vi "Auto Intake Mode.vi"(7 "Intake Angle":dbl, 11 "Intake Commands Cluster":T2={"Intake Commands"=enum."Load", "Intake Mode"=enum."Auto", "Override IR"=FALSE}) -> (0 "Intake States":T1, 2 "Roller Power":dbl, 3 "Angle Power":dbl, 4 "Target Height":dbl, 5 "Encoder Position":dbl, 6 "Rollers Active?":bool)   [LabVIEW 2015]
uses:
  Common Code/Intake Commands Cluster.ctl
  Common Code/Intake Commands.ctl
  Common Code/Intake Mode.ctl
  Common Code/Intake States.ctl
  Common Code/Change Detect Int.vi
  Common Code/Change Detect Double.vi
  Robot Global Data.vi
  <vilib>/addons/control/pid/pid.llb/PID (DBL).vi
  <vilib>/addons/control/pid/NI_PID_pid.lvlib
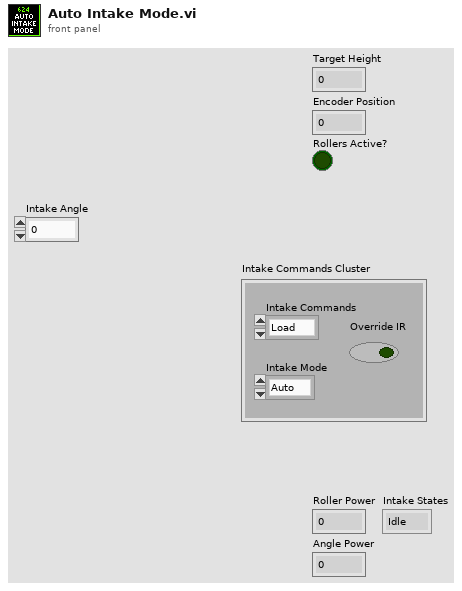
[diagram p1: front panel]
types:
  T1 = typedef "Intake States.ctl" = enum16{"Idle", "Set roller speed", "Move to angle"}
  T2 = typedef "Intake Commands Cluster.ctl" = cluster{"Intake Commands":T3, "Intake Mode":T4, "Override IR":bool}
  T3 = typedef "Intake Commands.ctl" = enum16{"Unload", "Load", "Pull up", "Drop low", "Idle", "Lift Half"}
  T4 = typedef "Intake Mode.ctl" = enum16{"Safe", "Auto", "Manual"}
  T5 = typedef "Dashboard Control Data.ctl" = cluster{"Shooter Presets":T6, "Encoder Control":T8, "Steer PID output":cluster{"output high":dbl, "output low":dbl}, " Steer PID gains":cluster{"proportional gain (Kc)":dbl, "integral time (Ti, min)":dbl, "derivative time (Td, min)":dbl}, "Drivetrain Settings":T9, "Vision Packet":T10, "Dashboard Drivetrain Command":T11, "Info/Command Cluster":T13, "Ball Vision Packet":T14, "Intake Presets":T16, "Intake Encoder Control":T18, "Climb Presets":T19, "Goal Output Range":cluster{"output high":dbl, "output low":dbl}, "Enabled Systems":T20, "Auton Presets":T21, "Pressure M":dbl, "Pressure B":dbl}
  T6 = typedef "Shooter Presets.ctl" = cluster{"Batter Shot":T7, "Deep Middle Shot":T7, "Manual Shot":T7, "Left Ticks Per Rotation":dbl, "Right Ticks Per Rotation":dbl, "Low Bar Shot":T7, "Shooter RPM Tolerance":dbl, "IIR Filter Power":dbl, "Trigger Power":dbl, "Fire from Load Delay":i32, "Max Angle":dbl, "Min Angle":dbl, "Angle PID gains":cluster{"P":dbl, "I":dbl, "D":dbl}, "Angle Output":cluster{"output high":dbl, "output low":dbl}, "Shooter Angle Tolerance":dbl, "Vision Shoot x^2":dbl, "Vision Shoot x":dbl, "Axis Camera Offset":dbl, "High Goal Center Height":dbl, "Feed Forward Max Accel":dbl, "Feed Forward Kv":dbl, "Backwards Trigger":dbl, "Shot Finish Delay (ms)":dbl, "Angle Max Current":dbl, "Angle Current Trip Time":dbl, "Intake Angle":dbl, "Vision Shoot c":dbl, "Reset?":bool, "Servo Release Delay":dbl, "Servo Idle Angle":i32, "Servo Hold Angle":i32, "Angle Pot x":dbl, "Angle Pot c":dbl, "Ignore Angle?":bool, "Manual Output?":bool, "Manual Out":dbl, "Max RPM":dbl, "Safty Frist Angle":dbl, "Intake Danger Height":dbl, "Angle Pot B":i32, "Angle Pot M":dbl, "FF Finish RPM":dbl, "RPM PID Right":cluster{"P":dbl, "I":dbl, "D":dbl, "FF":dbl}, "RPM PID Left":cluster{"P":dbl, "I":dbl, "D":dbl, "FF":dbl}, "Backwards RPM":dbl, "Vision RPM":dbl}
  T7 = typedef "Shot Presets.ctl" = cluster{"Left":dbl, "Right":dbl, "Angle":dbl}
  T8 = typedef "Encoder Control.ctl" = cluster{"Right Tick Constant":dbl, "Left Tick Constant":dbl, "Reset?":bool, "Y Dist":cluster{"PID gains":cluster{"proportional gain (Kc)":dbl, "integral time (Ti, min)":dbl, "derivative time (Td, min)":dbl}}, "Y Stop Thresh":dbl, "Y Stop Speed":dbl}
  T9 = typedef "Drivetrain Settings.ctl" = cluster{"Gyro Tolerance":dbl, "Throttle Ramp (ms)":dbl, "Angular rate compensation":bool, "Throttle to Rate Scale":dbl, "Rate compensation gain":dbl, "Kv":dbl, "Ka":dbl, "Feed Forward P":dbl, "Feed Forward D":dbl, "Goal Vision PID gains":cluster{"proportional gain (Kc)":dbl, "integral time (Ti, min)":dbl, "derivative time (Td, min)":dbl}, "Goal Detection Window":dbl, "Creep Rate":dbl}
  T10 = typedef "Goal Vision Packet.ctl" = cluster{"Distance":dbl, "Center X":dbl, "Center Y":dbl, "Found Target?":bool, "Robot Center":dbl, "Angle":dbl}
  T11 = typedef "Dashboard Drivetrain Command.ctl" = cluster{"Drivetrain Vision":T12}
  T12 = typedef "Drivetrain Vision.ctl" = cluster{"Goal Window":dbl, "Ball Window":dbl}
  T13 = typedef "Ball Tracking Command Cluster.ctl" = cluster{"Distance to Ball":dbl, "Desired Angle":dbl, "Command":enum16{"Turn to Ball", "Turn to Angle", "Get Distance"}, "Pixels from Center":dbl}
  T14 = typedef "Ball Vision Packet.ctl" = cluster{"Ball Detected?":bool, "Distance to Ball":dbl, "Desired Angle":dbl, "Pixels from Center":dbl, "Tracking mode":T15}
  T15 = typedef "Tracking Mode.ctl" = enum16{"Turn to Ball", "Turn to Angle"}
  T16 = typedef "Intake Presets.ctl" = cluster{"Intake Speed":dbl, "Outake Speed":dbl, "Low Height":dbl, "Half Height":dbl, "Full Height":dbl, "Angle Speed":dbl, "Angle Tolerance":dbl, "Encoder Scale":dbl, "Load Height":dbl, "Output Range":T17, "Rotation Power Max/Min":dbl, "MaxCurrent":dbl, "Intake Trip Time":dbl, "Idle Height":dbl, "Max Height":dbl, "Reset Encoders?":bool, "PID gains":cluster{"proportional gain (Kc)":dbl, "integral time (Ti, min)":dbl, "derivative time (Td, min)":dbl}}
  T17 = typedef "Drivetrain Output Range.ctl" = cluster{"output high":dbl, "output low":dbl}
  T18 = typedef "IntakeEcoderControl.ctl" = cluster{"Arm Tick Constant":dbl, "Reset?":bool, "Y Dist":cluster{"PID gains":cluster{"proportional gain (Kc)":dbl, "integral time (Ti, min)":dbl, "derivative time (Td, min)":dbl}}, "Y Stop Thresh":dbl, "Y Stop Speed":dbl}
  T19 = typedef "Climb Presets.ctl" = cluster{"Pull Power":dbl, "Time to Hold":dbl, "Extend Power":dbl}
  T20 = typedef "Enabled Systems.ctl" = cluster{"Shoot":bool, "Intake":bool, "DT":bool, "Gyro":bool, "100ms":bool, "US":bool}
  T21 = typedef "Autonomous Presets.ctl" = cluster{"Pitch Limit":dbl, "Roll Limit":dbl, "Ultrasonic Limit":dbl, "Start Position":dbl, "Cross Position":dbl}
  T22 = cluster{"proportional gain (Kc)":dbl, "integral time (Ti, min)":dbl, "derivative time (Td, min)":dbl}
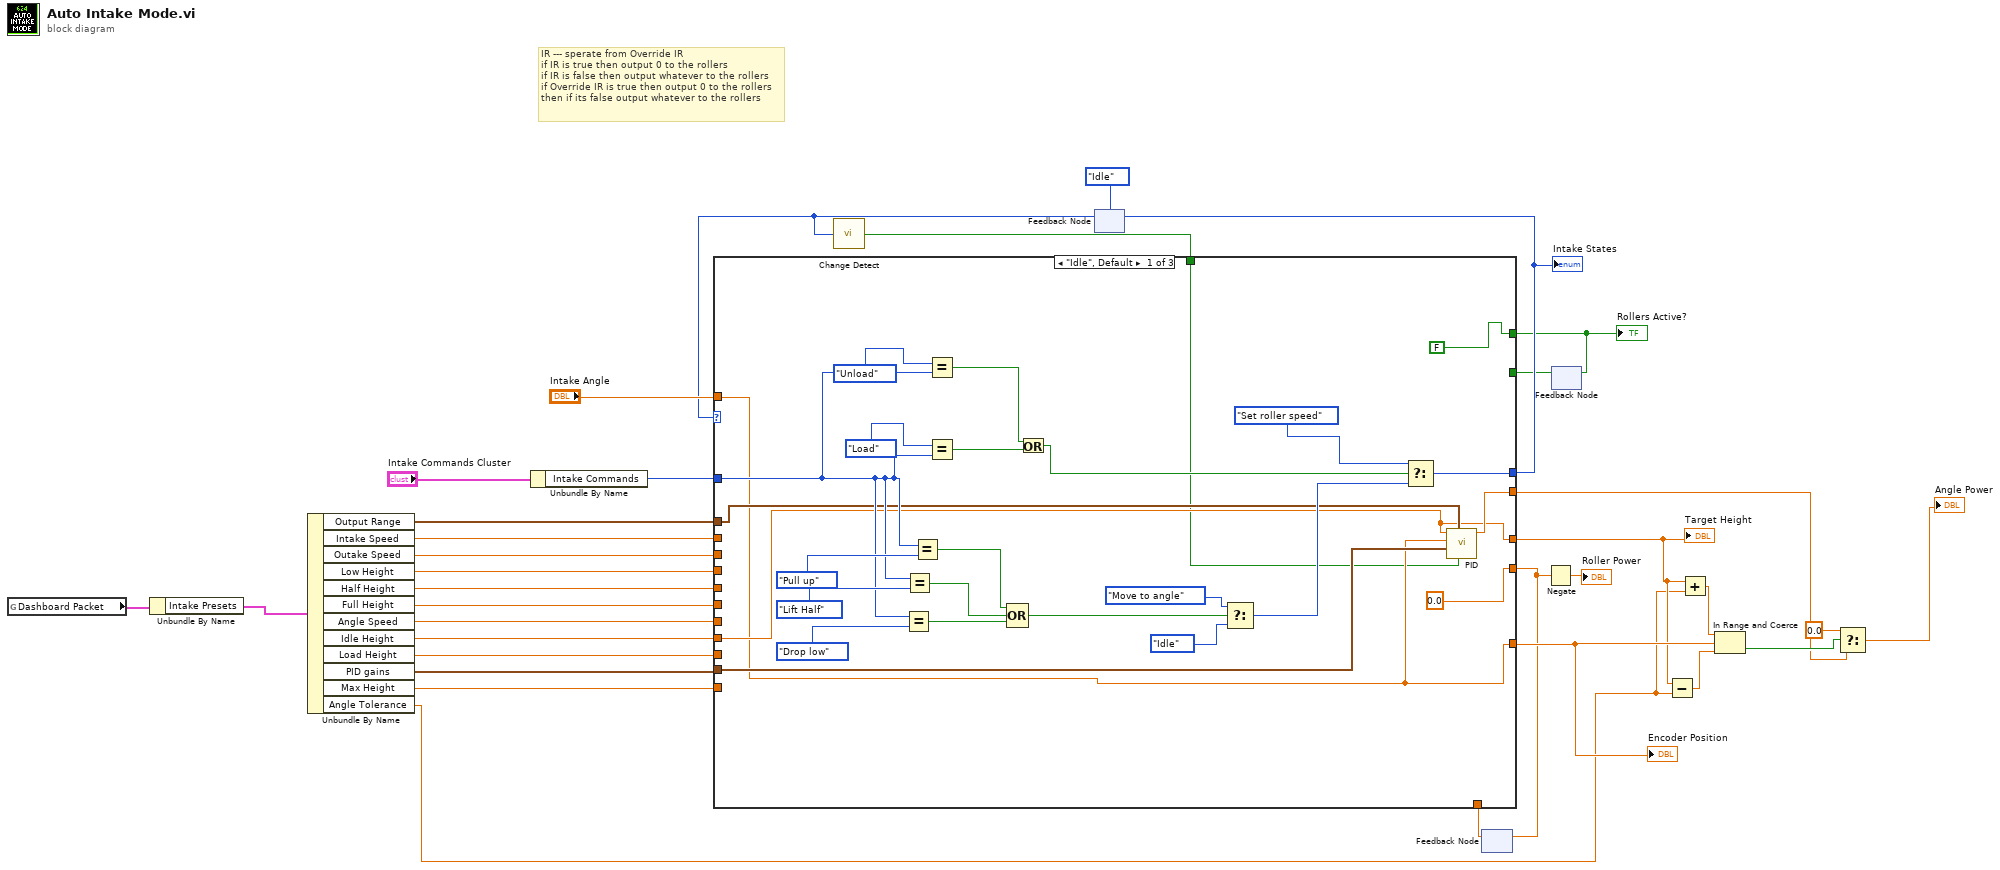
[diagram p0: block diagram]
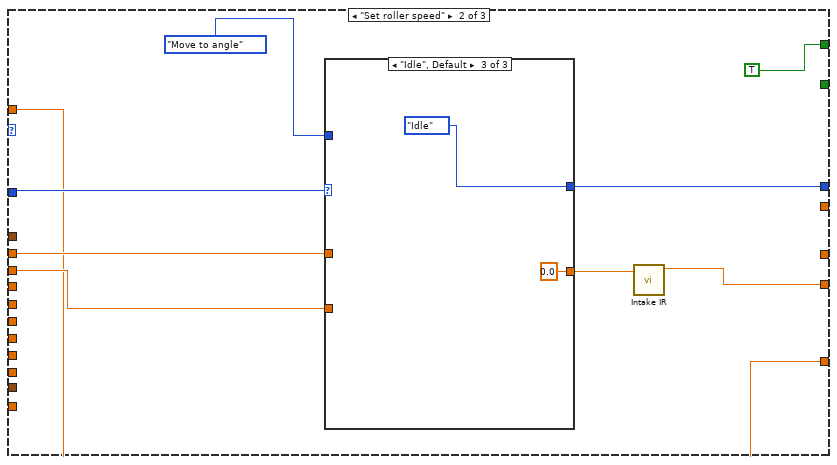
[diagram p2: hidden frame]
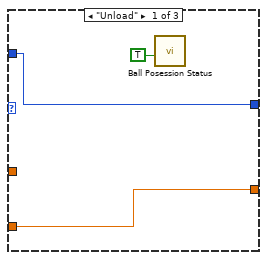
[diagram p3: hidden frame]
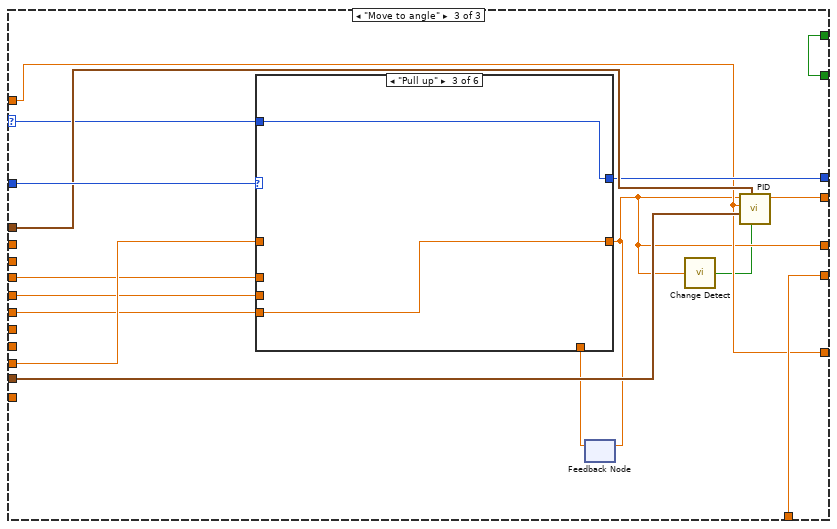
[diagram p5: hidden frame]
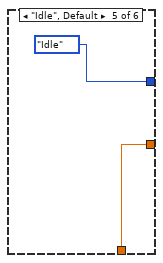
[diagram p9: hidden frame]
diagram:
  # "IR --- sperate from Override IR \nif IR is true then output 0 to the rollers\nif IR is false then output whatever to the rollers\nif Override IR is true then output 0 to the rollers\nthen if its false output whatever to the rollers"
  n1 = global read "Robot Global Data.vi" "Dashboard Packet"() -> (w16:T5)
  n2 = Unbundle By Name(w16) -> ("Intake Presets"=w17:T16)
  n3 = Unbundle By Name(w17) -> ("Output Range"=w27:T17, "Intake Speed"=w26:dbl, "Outake Speed"=w25:dbl, "Low Height"=w24:dbl, "Half Height"=w23:dbl, "Full Height"=w22:dbl, "Angle Speed"=w21:dbl, "Idle Height"=w20:dbl, "Load Height"=w19:dbl, "PID gains"=w18:T22, "Max Height"=w15:dbl, "Angle Tolerance"=w12:dbl)
  n4 = Unbundle By Name("Intake Commands Cluster") -> ("Intake Commands"=w32:T3)
  n5 = feedback #1(Intake_States."Idle") -> (w5:T1)
  n6 = call-poly "Change Detect.vi"("In"=w5) -> ("Changed?"=w4:bool)
  n7 = feedback #2() -> (w30:dbl)  [unwired: 1 in]
  n8 = feedback #3() -> (w28:bool)  [unwired: 1 in]
  n9 = case shown="\"Idle\", Default" w5 {
    selector: w5 -> [_ _ w80]
    tunnel: w32 -> [w46 w69 w92]
    tunnel: [w50 w67 w81] -> w31
    tunnel: w27 -> [w40 _ w84]
    tunnel: w25 -> [_ w65 _]
    tunnel: w22 -> [_ _ w87]
    tunnel: w26 -> [_ w66 _]
    tunnel: w23 -> [_ _ w89]
    tunnel: w21 -> [_ _ _]
    tunnel: w24 -> [_ _ w88]
    tunnel: [0.0 ("Intake Speed") w63 w91] -> w3
    tunnel: w30 -> [_ _ w91]
    tunnel: w19 -> [_ _ w90]
    tunnel: [w39 _ w86] -> w1
    tunnel: "Intake Angle" -> [w36 w61 w79]
    tunnel: w18 -> [w41 _ w85]
    tunnel: w20 -> [w38 _ _]
    tunnel: [w38 _ w78] -> w13
    tunnel: [w36 w61 w79] -> w14
    tunnel: [FALSE TRUE w82] -> w29
    tunnel: w28 -> [_ _ w82]
    tunnel: w15 -> [_ _ _]
    tunnel: w4 -> [w35 _ _]
    frame "Idle", Default {
      n10 = Equal?(x=w46, y=Intake_Commands."Drop low" ("Intake Commands")) -> (x = y?=w52:bool)
      n11 = Equal?(x=w46, y=Intake_Commands."Lift Half" ("Intake Commands")) -> (x = y?=w53:bool)
      n12 = Equal?(x=w46, y=Intake_Commands."Pull up" ("Intake Commands")) -> (x = y?=w57:bool)
      n13 = Equal?(x=Intake_Commands."Unload" ("Intake Commands"), y=w46) -> (x = y?=w45:bool)
      n14 = Equal?(x=Intake_Commands."Load" ("Intake Commands"), y=w46) -> (x = y?=w44:bool)
      n15 = Compound Arithmetic op=OR(w57, w53, w52) -> (w56:bool)
      n16 = Or(x=w45, y=w44) -> (x .or. y?=w43:bool)
      n17 = Select(t=Intake_States."Move to angle", s=w56, f=Intake_States."Idle") -> (s? t:f=w51:T1)
      n18 = Select(t=Intake_States."Set roller speed", s=w43, f=w51) -> (s? t:f=w50:T1)
      n19 = call-poly <vilib>:"PID.vi"("reinitialize? (F)"=w35, "output range"=w40, "PID gains"=w41, "process variable"=w36, "setpoint"=w38) -> ("output"=w39:dbl)  [unwired: 5 in, 1 out]
    }
    frame "Set roller speed" {
      n20 = case shown="\"Idle\", Default" w69 {
        tunnel: Intake_States."Move to angle" -> [w72 w74 _]
        tunnel: [w72 w74 Intake_States."Idle"] -> w67
        tunnel: w66 -> [_ w73 _]
        tunnel: [w71 w73 0.0 ("Intake Speed")] -> w62
        tunnel: w65 -> [w71 _ _]
        frame "Unload" {
          n21 = call "Ball Posession Status.vi"("Logical Exit?"=TRUE) -> ()  [unwired: 10 in, 1 out]
        }
        frame "Load" {
        }
        frame "Idle", Default {
        }
      }
      n22 = call "Intake IR.vi"("Speed"=w62) -> ("Speeeeeeed"=w63:dbl)  [unwired: 10 in]
    }
    frame "Move to angle" {
      n23 = feedback #4() -> (w83:dbl)  [unwired: 1 in]
      n24 = case shown="\"Pull up\"" w92 {
        tunnel: w90 -> [w94 w96 _ _ _ _]
        tunnel: [w94 w96 w98 w100 w102 w104] -> w78
        tunnel: w89 -> [_ _ _ _ _ w104]
        tunnel: w88 -> [_ _ _ w100 _ _]
        tunnel: w87 -> [_ _ w98 _ _ _]
        tunnel: w83 -> [_ _ _ _ w102 _]
        tunnel: [w93 w95 w97 w99 Intake_States."Idle" w103] -> w81
        tunnel: w80 -> [w93 w95 w97 w99 _ w103]
        frame "Unload" {
        }
        frame "Load" {
        }
        frame "Pull up" {
        }
        frame "Drop low" {
        }
        frame "Idle", Default {
        }
        frame "Lift Half" {
        }
      }
      n25 = feedback-in #4(w78) -> ()
      n26 = call-poly "Change Detect.vi"("In"=w78) -> ("Changed?"=w77:bool)
      n27 = call-poly <vilib>:"PID.vi"("reinitialize? (F)"=w77, "output range"=w84, "PID gains"=w85, "process variable"=w79, "setpoint"=w78) -> ("output"=w86:dbl)  [unwired: 5 in, 1 out]
    }
  }
  "Intake States" <- w31
  "Target Height" <- w13
  "Encoder Position" <- w14
  "Rollers Active?" <- w29
  n28 = feedback-in #1(w31) -> ()
  n29 = feedback-in #2(w3) -> ()
  n30 = Negate(x=w3) -> (-x=→"Roller Power":dbl)
  n31 = feedback-in #3(w29) -> ()
  n32 = Subtract(x=w13, y=w12) -> (x-y=w11:dbl)
  n33 = Add(x=w13, y=w12) -> (x+y=w10:dbl)
  n34 = In Range and Coerce(upper limit=w10, x=w14, lower limit=w11) -> (In Range?=w9:bool)  [unwired: 1 out]
  n35 = Select(t=0.0, s=w9, f=w1) -> (s? t:f=→"Angle Power":dbl)
